vi "Get Connections - NPin MConn.vi"(6 "pin type":T1, 8 "error in":errorcluster, 9 "site":i32=-1, 10 "pin or relay names":string[](array[string]), 11 "session reservation in":refnum<class "Session Reservation.lvclass">) -> (0 "error out":errorcluster, 2 "connections":T2[](array[typedef]), 3 "session reservation out":refnum<class "Session Reservation.lvclass">)   [LabVIEW 2020, in "MeasurementLink niFGEN.lvlib"]
doc: "Gets the NI-FGEN connection information for the given <b>pin type</b>, <b>pin or relay names</b>, and <b>site</b>. If the <b>pin or relay names</b> input is unwired, the connection information for all pins for the given <b>site</b> will be returned. If the <b>site</b> input is unwired, the connection information for the given <b>pin or relay names</b> for all sites will be returned. If both the <b>pin or relay names</b> and <b>site</b> inputs are unwired, the connection information for all pins and all sites will be returned.\n\nIf you have not called <b>Create Sessions.vi</b> prior to calling this VI, the connection information will be returned with the correct information but will have an invalid session."
uses:
  MeasurementLink niFGEN.lvlib
  MeasurementLink Session Management/Session Reservation/Connection.ctl
  MeasurementLink Session Management/Session Reservation/Session Reservation.lvclass
  Connection with Session.ctl
  1016b550-acf3-415d-ab7a-971f7ba5cd11.vi
  Instrument/Instrument.lvclass
  MeasurementLink Session Management/Session Reservation/Pin Type.ctl
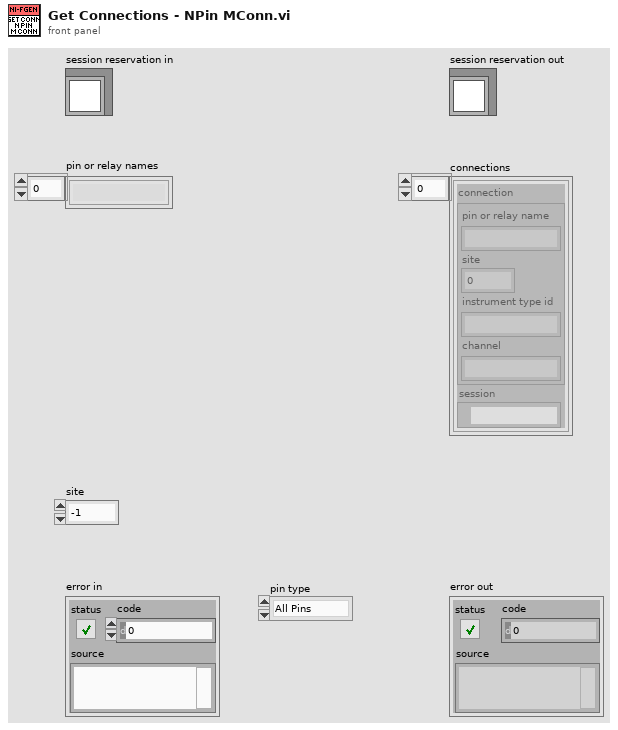
[diagram p1: front panel]
types:
  T1 = typedef "MeasurementLink Session Management.lvlib/Session Reservation.lvclass/Pin Type.ctl" = enum16{"All Pins", "DUT Pins", "System Pins"}
  T2 = typedef "MeasurementLink niFGEN.lvlib/Connection with Session.ctl" = cluster{"connection":T3, "session":refnum<k15>}
  T3 = typedef "MeasurementLink Session Management.lvlib/Session Reservation.lvclass/Connection.ctl" = cluster{"pin or relay name":string, "site":i32, "instrument type id":string, "channel":string}
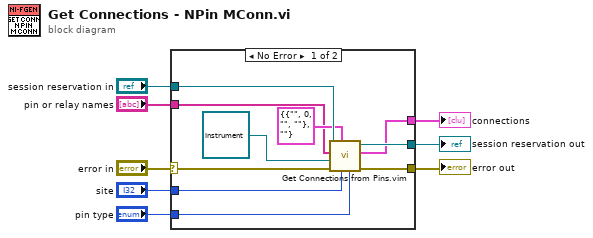
[diagram p0: block diagram]
diagram:
  n1 = case shown="No Error" "error in" {
    selector: "error in" -> [w11 w19]
    tunnel: "session reservation in" -> [w15 w20]
    tunnel: "pin or relay names" -> [w12 _]
    tunnel: [w16 w19] -> w5
    tunnel: [w18 w20] -> w4
    tunnel: [w17 _] -> w3
    tunnel: "site" -> [w14 _]
    tunnel: "pin type" -> [w9 _]
    frame No Error {
      n2 = call "Get Connections from Pins.vim"("pin type"=w9, "site"=w14, "connection type"=T2 {"connection"={"pin or relay name"="", "site"=0, "instrument type id"="", "channel"=""}, "session"=""} ("niDCPower connection"), "error in"=w11, "instrument"=refnum<class "Instrument.lvclass"> refnum ("MeasurementLink niFGEN.lvlib:Instrument.lvclass"), "pin or relay names"=w12, "session reservation in"=w15) -> ("error out"=w16:errorcluster, "connections"=w17:T2[], "session reservation out"=w18:refnum<class "Session Reservation.lvclass">)  [unwired: 2 in]
    }
    frame Error {
    }
  }
  "error out" <- w5
  "session reservation out" <- w4
  "connections" <- w3
